vi "LocalFileName.vi"(1 "file name":string, 2 "VI path":path) -> (0 "full path":path)   [LabVIEW 2009]
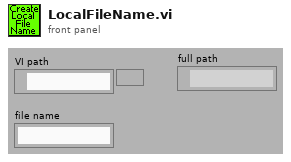
[diagram p1: front panel]
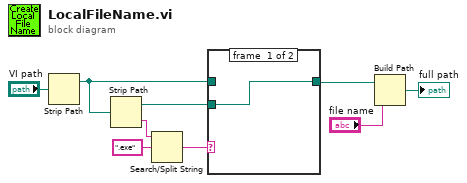
[diagram p0: block diagram]
diagram:
  n1 = Strip Path(path="VI path") -> (stripped path=w9:path)  [unwired: 1 out]
  n2 = Strip Path(path=w9) -> (stripped path=w3:path, name=w8:string)
  n3 = Search/Split String(string=w8, search string/char (-)=".exe") -> (match + rest of string=w6:string)  [unwired: 1 in, 2 out]
  n4 = case shown="\".exe\"" w6 {
    tunnel: w9 -> [_ w11]
    tunnel: [w10 w11] -> w2
    tunnel: w3 -> [w10 _]
    frame #0 {
    }
    frame #1 {
    }
  }
  n5 = Build Path(base path=w2, name or relative path="file name") -> (appended path=→"full path":path)
